vi "FTW-CodeGen-Initialize.vi"(5 "XRef":refnum<vi>) -> (4 "State Out":T1)   [LabVIEW 2012, in "FTW-JSON-Serialize.xnode"]
uses:
  FTW-JSON-Serialize.xnode
  FTW-CodeGen-State.ctl
panel:
  # "Inputs"
  # "Outputs"
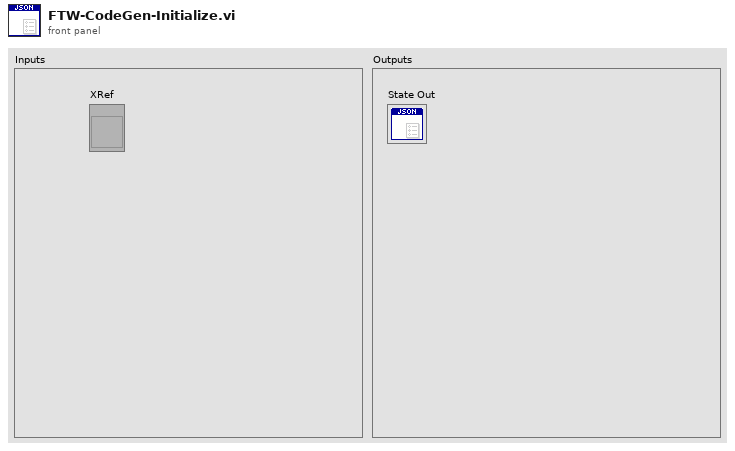
[diagram p1: front panel]
types:
  T1 = typedef "FTW-JSON-Serialize.xnode/FTW-CodeGen-State.ctl" = cluster{"Prototype Filepath":path}
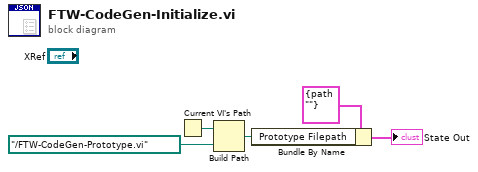
[diagram p0: block diagram]
diagram:
  n1 = Current VI's Path() -> (path=w5:path)
  n2 = Build Path(base path=w5, name or relative path=path "../FTW-CodeGen-Prototype.vi") -> (appended path=w1:path)
  n3 = Bundle By Name(cluster=T1 {"Prototype Filepath"=path ""} ("State"), "Prototype Filepath"=w1) -> (→"State Out":T1)
